vi "Network control test 1.vi"() -> ()   [LabVIEW 2016]
uses:
  <vilib>/Utility/miscctls.llb/LVPointTypeDef.ctl
panel:
  out "shared variable refnum out":refnum<k21>
  out "SV set?":bool
  in  "Shared Variable":refnum<k21>="ni.var.psp://localhost/Shared_Variables/Network-shared string variable"
  in  "Sync":bool
  out "Received string":string
  in  "Type string":string
  in  "Stop":bool
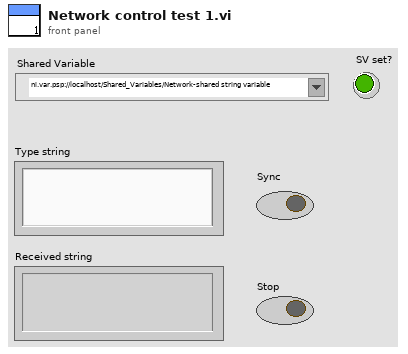
[diagram p1: front panel]
types:
  T1 = typedef "LVPointTypeDef.ctl" = cluster{"Horizontal":i16, "Vertical":i16}
  T2 = cluster{"Read Access":enum8{"Allowed", "Required", "None"}, "Write Access":enum8{"Allowed", "Required", "None"}}
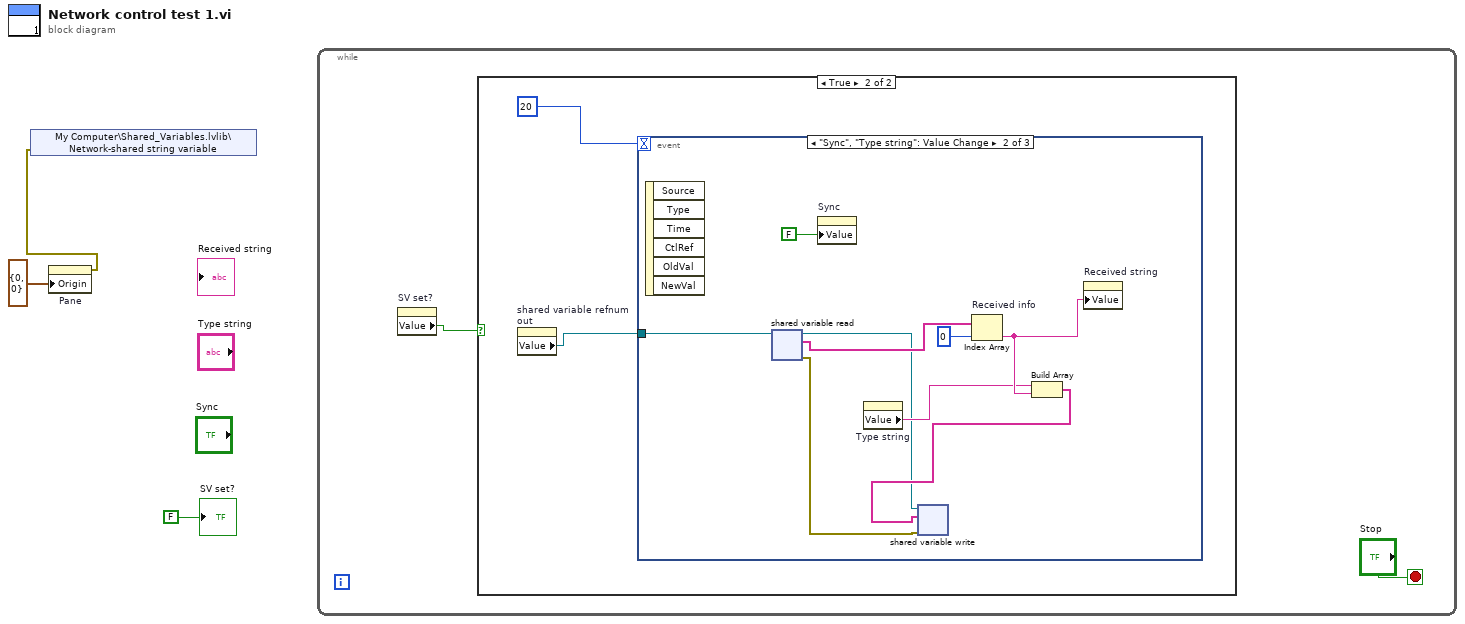
[diagram p0: block diagram]
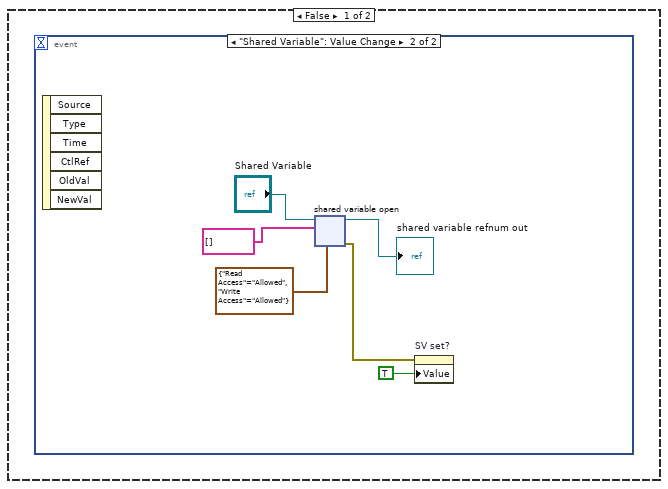
[diagram p2: hidden frame]
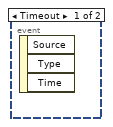
[diagram p3: hidden frame]
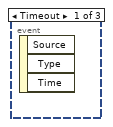
[diagram p4: hidden frame]
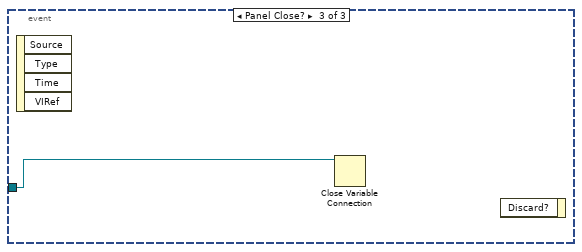
[diagram p5: hidden frame]
diagram:
  n1 = property on="Pane" class="Pane"("Origin"=T1 {"Horizontal"=0, "Vertical"=0}) -> (error out=w1:errorcluster)  [unwired: 2 in, 1 out]
  n2 = shared-variable "My Computer\\Shared_Variables.lvlib\\Network-shared string variable"(error in=w1) -> ()  [unwired: 2 out]
  n3 = while {
    stop <- "Stop" stop-if-true
    n4 = property on="SV set?" class="Bool (strict)"() -> ("Value"=w4:bool)  [unwired: 2 in, 2 out]
    n5 = case shown="True" w4 {
      frame False {
        n6 = event shown="[1] \"Shared Variable\": Value Change" {
          selector: _ -> [_ _]
          dyn-events: _ -> [_ _]
          timeout: _ -> [_ _]
          event Timeout {
            n7 = event-data() -> ()  [unwired: 1 in, 3 out]
          }
          event "Shared Variable": Value Change {
            n8 = event-data() -> ()  [unwired: 1 in, 6 out]
            n9 = shared-variable-open("Shared Variable", string[] [] ("appended array"), T2 {"Read Access"=enum."Allowed", "Write Access"=enum."Allowed"} ("access")) -> (→"shared variable refnum out":refnum<k21>, w7:errorcluster)  [unwired: 1 in]
            n10 = property on="SV set?" class="Bool (strict)"(error in=w7, "Value"=TRUE ("SV set?")) -> ()  [unwired: 1 in, 2 out]
          }
        }
      }
      frame True {
        n11 = property on="shared variable refnum out" class="Variable (strict)"() -> ("Value"=w12:refnum<k21>)  [unwired: 2 in, 2 out]
        n12 = event shown="[1] \"Sync\", \"Type string\": Value Change" {
          selector: _ -> [_ _ _]
          dyn-events: _ -> [_ _ _]
          timeout: 20 -> [_ _ _]
          tunnel: w12 -> [_ w19 w23]
          event Timeout {
            n13 = event-data() -> ()  [unwired: 1 in, 3 out]
          }
          event "Sync", "Type string": Value Change {
            n14 = event-data() -> ()  [unwired: 1 in, 6 out]
            n15 = shared-variable-read(w19) -> (w14:refnum<k21>, w15:errorcluster, w18:string[])  [unwired: 1 in, 1 out]
            n16 = property on="Sync" class="Bool (strict)"("Value"=FALSE ("Sync")) -> ()  [unwired: 2 in, 2 out]
            n17 = property on="Type string" class="Str"() -> ("Value"=w20:string)  [unwired: 2 in, 2 out]
            n18 = Index Array "Received info"(array=w18, index=0) -> (element=w21:string)
            n19 = Build Array(w20, w21) -> (w16:string[])
            n20 = shared-variable-write(w14, w15, w16) -> ()  [unwired: 2 out]
            n21 = property on="Received string" class="Str"("Value"=w21) -> ()  [unwired: 2 in, 2 out]
          }
          event Panel Close? {
            n22 = event-data() -> ()  [unwired: 1 in, 4 out]
            n23 = Close Variable Connection(11:w23) -> ()  [unwired: 1 in, 1 out]
            n24 = event-data() -> ()  [unwired: 2 in, 1 out]
          }
        }
      }
    }
  }
  "SV set?" <- FALSE ("SV set?")
